vi "niRFUtil MASMT Util Get Resample State Info Type.vi"(1 "resample state info in":T1 {"extractFilterMethod" items=["Interpolation", "Rounding"]}) -> (0 "resample state info out":T1 {"extractFilterMethod" items=["Interpolation", "Rounding"]})   [LabVIEW 2015, in "niRFUtil.lvlib"]
uses:
  niRFUtil.lvlib
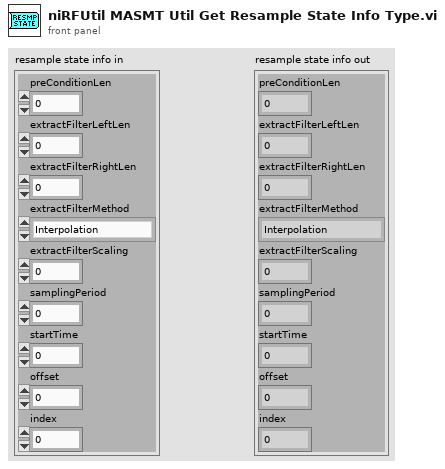
[diagram p1: front panel]
types:
  T1 = cluster{"preConditionLen":i32, "extractFilterLeftLen":i32, "extractFilterRightLen":i32, "extractFilterMethod":i32, "extractFilterScaling":dbl, "samplingPeriod":dbl, "startTime":dbl, "offset":dbl, "index":i32}
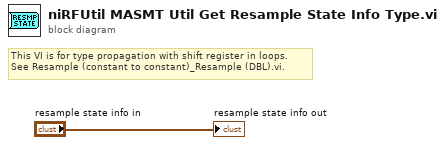
[diagram p0: block diagram]
diagram:
  # "This VI is for type propagation with shift register in loops.\nSee Resample (constant to constant)_Resample (DBL).vi."
  "resample state info out" <- "resample state info in"
